vi "SingleWaveformProbe.vi"() -> ()   [LabVIEW 2010]
panel:
  in  "Probe":waveform(dbl)
  out "Waveform Graph":waveform(dbl)(graph)
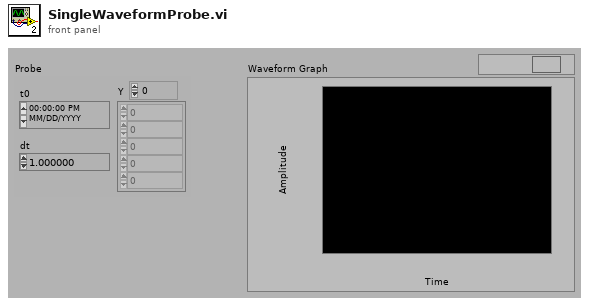
[diagram p1: front panel]
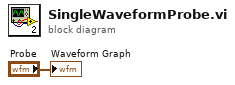
[diagram p0: block diagram]
diagram:
  "Waveform Graph" <- "Probe"
